vi "COMI INT Get Int Chan.vi"(7 "nMode":i32, 9 "nState":i32, 10 "NumCh":i32, 11 "hDevice":u32) -> (1 "nState out":i32, 2 "function return":i32, 3 "hDevice out":u32, 5 "nMode out":i32)   [LabVIEW 2017, in "Comidll.lvlib"]
doc: "long (COMI_INT_GetIntChan) (HANDLE hDevice, int NumCh, long *nState, long *nMode);"
uses:
  <userlib>/Comidll/Comidll.lvlib
  <userlib>/Comidll/Comidll.dll
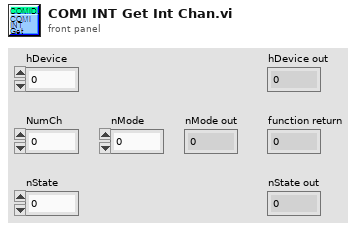
[diagram p1: front panel]
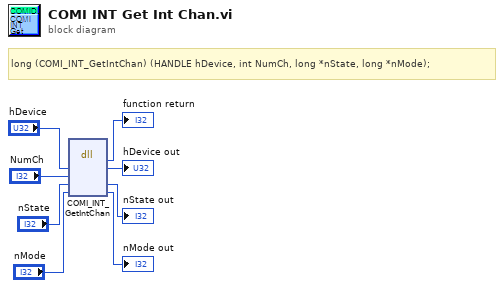
[diagram p0: block diagram]
diagram:
  # "long\t(COMI_INT_GetIntChan) (HANDLE hDevice, int NumCh, long *nState, long *nMode);"
  n1 = dll-call lib="C:/Program Files/National Instruments/LabVIEW 2017/user.lib/Comidll/Comidll.*" fn="COMI_INT_GetIntChan"("hDevice"="hDevice", "NumCh"="NumCh", "nState"="nState", "nMode"="nMode") -> (→"function return":i32, "hDevice"=→"hDevice out":u32, "nState"=→"nState out":i32, "nMode"=→"nMode out":i32)  [unwired: 4 in, 2 out]
